vi "Launcher.vi"() -> ()   [LabVIEW 2019, in "Project Sync Tools.lvclass"]
uses:
  Project Sync Tools.lvclass
panel:
  in  "Project Path":path
  out "Errors":errorcluster
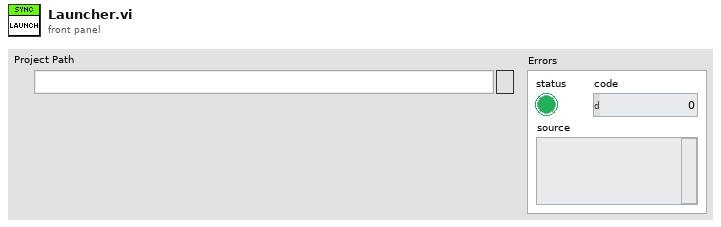
[diagram p1: front panel]
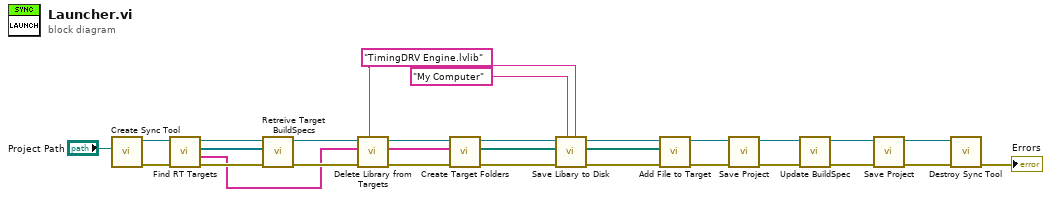
[diagram p0: block diagram]
diagram:
  w12 = "TimingDRV Engine.lvlib" ("Library Name")
  n1 = call "Create Sync Tool.vi"("File Path Control"="Project Path") -> ("error out"=w24:errorcluster, "CD Build Tools out"=w23:refnum<class "Project Sync Tools.lvclass">)  [unwired: 9 in]
  n2 = call "Find RT Targets.vi"("error in (no error)"=w24, "Project Sync Tools in"=w23) -> ("error out"=w25:errorcluster, "RT Targets names"=w5:string[], "RT Targets refs"=w26:refnum<vi>[], "Project Sync Tools out"=w27:refnum<class "Project Sync Tools.lvclass">)  [unwired: 6 in]
  n3 = call "Retreive Target BuildSpecs.vi"("error in (no error)"=w25, "Target Names in"=w26, "Project Sync Tools in"=w27) -> ("error out"=w6:errorcluster, "Project Sync Tools out"=w7:refnum<class "Project Sync Tools.lvclass">)  [unwired: 6 in, 1 out]
  n4 = call "Delete Library from Targets.vi"("Library Name"=w12, "error in (no error)"=w6, "Target Names in"=w5, "Project Sync Tools in"=w7) -> ("error out"=w21:errorcluster, "Target Names out"=w14:string[], "Project Sync Tools out"=w22:refnum<class "Project Sync Tools.lvclass">)  [unwired: 5 in]
  n5 = call "Create Target Folders.vi"("error in (no error)"=w21, "Target Names in"=w14, "Project Sync Tools in"=w22) -> ("error out"=w18:errorcluster, "RT Targets Folders"=w19:path[], "Project Sync Tools out"=w20:refnum<class "Project Sync Tools.lvclass">)  [unwired: 6 in]
  n6 = call "Save Libary to Disk.vi"("Library Name"=w12, "Target Name"="My Computer", "error in (no error)"=w18, "Destination Directories"=w19, "Project Sync Tools in"=w20) -> ("error out"=w16:errorcluster, "New Library Paths"=w15:path[], "Project Sync Tools out"=w17:refnum<class "Project Sync Tools.lvclass">)  [unwired: 4 in]
  n7 = call "Add File to Target.vi"("error in (no error)"=w16, "Target Name"=w15, "Project Sync Tools in"=w17) -> ("error out"=w4:errorcluster, "Project Sync Tools out"=w3:refnum<class "Project Sync Tools.lvclass">)  [unwired: 7 in]
  n8 = call "Save Project.vi"("error in (no error)"=w4, "Project Sync Tools in"=w3) -> ("error out"=w1:errorcluster, "Project Sync Tools out"=w2:refnum<class "Project Sync Tools.lvclass">)  [unwired: 8 in]
  n9 = call "Update BuildSpec.vi"("error in (no error)"=w1, "CD Build Tools in"=w2) -> ("error out"=w11:errorcluster, "CD Build Tools out"=w10:refnum<class "Project Sync Tools.lvclass">)  [unwired: 8 in]
  n10 = call "Save Project.vi"("error in (no error)"=w11, "Project Sync Tools in"=w10) -> ("error out"=w9:errorcluster, "Project Sync Tools out"=w8:refnum<class "Project Sync Tools.lvclass">)  [unwired: 8 in]
  n11 = call "Destroy Sync Tool.vi"("error in (no error)"=w9, "CD Build Tools in"=w8) -> ("error out"=→"Errors":errorcluster)  [unwired: 9 in]
